vi "Set Caller Enqueuer.vi"(8 "error in (no error)":errorcluster, 10 "Caller Enqueuer":refnum<class "Message Enqueuer.lvclass">, 11 "Open Form Button in":refnum<class "Open Form Button.lvclass">) -> (0 "error out":errorcluster, 3 "Open Form Button out":refnum<class "Open Form Button.lvclass">)   [LabVIEW 2020, in "Panel Form Controller.lvlib" / "Open Form Button.lvclass"]
uses:
  Open Form Button.lvclass
  <vilib>/ActorFramework/Message Enqueuer/Message Enqueuer.lvclass
  Open Form Button.lvclass/Open Form Button.ctl
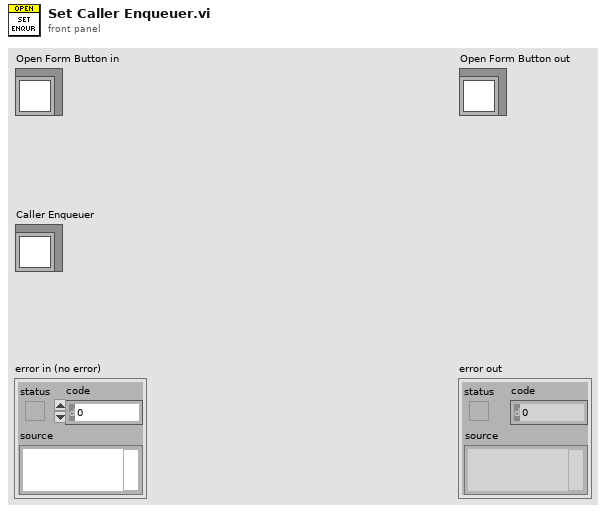
[diagram p1: front panel]
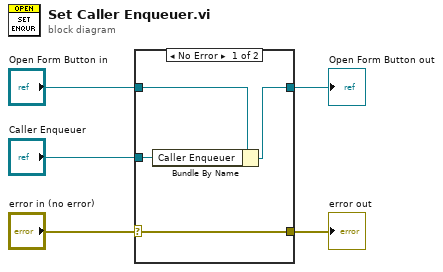
[diagram p0: block diagram]
diagram:
  n1 = case shown="No Error" "error in (no error)" {
    selector: "error in (no error)" -> [w9 w11]
    tunnel: [w9 w11] -> w4
    tunnel: [w7 w10] -> w2
    tunnel: "Open Form Button in" -> [w8 w10]
    tunnel: "Caller Enqueuer" -> [w6 _]
    frame No Error {
      n2 = Bundle By Name(cluster=w8, "Caller Enqueuer"=w6) -> (w7:refnum<class "Open Form Button.lvclass">)
    }
    frame Error {
    }
  }
  "error out" <- w4
  "Open Form Button out" <- w2
